vi "Wait Until Not Busy on Device.vi"(8 "error in (no error)":errorcluster, 11 "cluster of private data in":T1={"FPGA VI Reference"=refnum, "device index"=0, "screen size"=enum."8x1", "font size"=enum."5x8", "auto wrap"=FALSE, "alignment"=enum."None", "number of line"=enum."2 lines", "shift 0"=0, "entry mode 0"=enum."increment & no shift", "shift 1"=0, "entry mode 1"=enum."increment & no shift"}) -> (0 "error out":errorcluster, 3 "cluster of private data out":T1={"FPGA VI Reference"=refnum, "device index"=0, "screen size"=enum."8x1", "font size"=enum."5x8", "auto wrap"=FALSE, "alignment"=enum."None", "number of line"=enum."2 lines", "shift 0"=0, "entry mode 0"=enum."increment & no shift", "shift 1"=0, "entry mode 1"=enum."increment & no shift"})   [LabVIEW 2017, in "HD44780.lvclass"]
uses:
  HD44780.lvclass
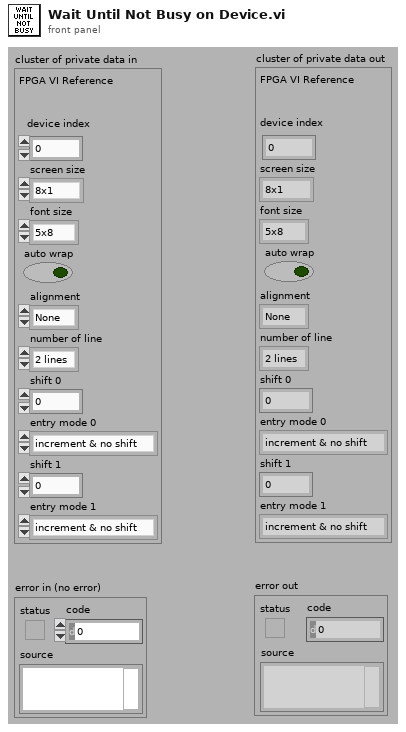
[diagram p1: front panel]
types:
  T1 = cluster{"FPGA VI Reference":refnum<k20>, "device index":i8, "screen size":enum8{"8x1", "8x2", "12x4", "16x1", "16x2", "16x4", "20x1", "20x2", "20x4", "24x1", "24x2", "40x2", "40x4"}, "font size":enum8{"5x8", "5x10"}, "auto wrap":bool, "alignment":enum16{"None", "Left", "Center", "Right"}, "number of line":enum8{"1 line", "2 lines"}, "shift 0":i8, "entry mode 0":enum8{"increment & no shift", "increment & shift", "decrement & no shift", "decrement & shift"}, "shift 1":i8, "entry mode 1":enum8{"increment & no shift", "increment & shift", "decrement & no shift", "decrement & shift"}}
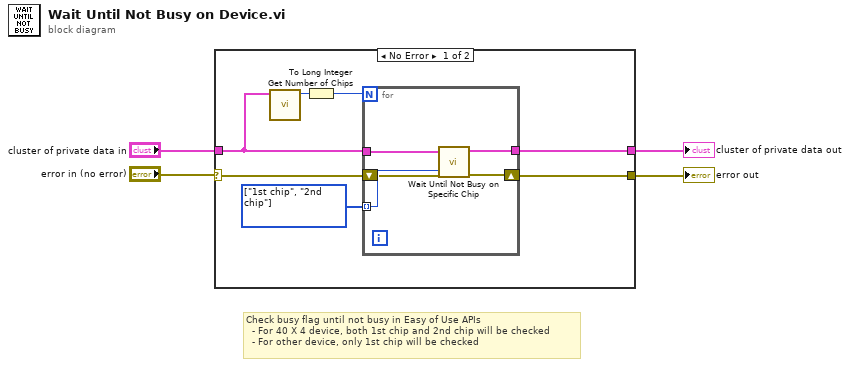
[diagram p0: block diagram]
diagram:
  # "Check busy flag until not busy in Easy of Use APIs\n  - For 40 X 4 device, both 1st chip and 2nd chip will be checked\n  - For other device, only 1st chip will be checked"
  n1 = case shown="No Error" "error in (no error)" {
    selector: "error in (no error)" -> [w9 w18]
    tunnel: [w10 w18] -> w4
    tunnel: "cluster of private data in" -> [w6 w17]
    tunnel: [w5 w17] -> w1
    frame No Error {
      w11 = enum16{"1st chip", "2nd chip"}[] [enum."1st chip", enum."2nd chip"] items=["1st chip", "2nd chip"] ("initialized array")
      n2 = call "Get Number of Chips.vi"("cluster of private data in"=w6) -> ("number of chips"=w8:u8)  [unwired: 10 in]
      n3 = To Long Integer(number=w8) -> (32bit integer=w7:i32)
      n4 = for {
        N: w7 -> [_]
        tunnel: w11 -> [w16] mode=indexing
        tunnel: w6 -> [w13]
        shift-right: [w15] -> w10
        shift-left: w9 -> [w14]
        tunnel: [w12] -> w5
        n5 = call "Wait Until Not Busy on Specific Chip.vi"("chip select  (1st chip)"=w16, "error in (no error)"=w14, "cluster of private data in"=w13) -> ("error out"=w15:errorcluster, "cluster of private data out"=w12:T1)  [unwired: 7 in]
      }
    }
    frame Error {
    }
  }
  "error out" <- w4
  "cluster of private data out" <- w1
